vi "add_mppt_data_to_log.vi"(0 "Experiment Indicator":string, 1 "Cell details cluster":T2={"Cell Position"=16, "Cell Label"="", "Pixel to measure"=0, "Area (cm^2)"=0.126, "Variable"="", "Variable value"="", "Scan settings in queue"=0, "Light or dark"="", "Measurement Type"=""} {"Pixel to measure" items=["All", "1", "2", "3", "4", "5", "6", "7", "8"]}, 3 "Intensity (no. of suns)":string, 4 "mppt folder path":path, 5 "mppt file path":path, 7 "Scan settings":T1={"J-V scan"=TRUE, "Start voltage (V)"=0.0, "End voltage (V)"=0.0, "Step voltage (V)"=1.4, "Scan both directions"=TRUE, "Inverted device structure"=FALSE, "Measurement delay (s)"=10.0, "Measurement speed"=0, "Scan rate (V/s)"=0.0, "Stabilisation time (s)"=0.0, "Stabilisation mode"=0, "Stabilisation value (V or A) "=1.0, "Illumination"=0, "Stabilisation in the dark?"=FALSE, "Repeat light scans"=FALSE, "No. of repeat scans"=0.0, "Only repeat for best pixel"=1, "J-t scan"=FALSE, "J-t best pixel only"=7, "J-t start voltage (V)"=0.0, "J-t end voltage (V)"=1.4, "J-t step voltage (V)"=0.01, "Step time (s)"=0.7, "J-t scan both directions"=TRUE, "J-t inverted device structure"=FALSE, "Settling delay (s)"=0.0, "J-t measurement speed"=0, "J-t illumination"=2, "Max. power stabilisation"=FALSE, "Max power best pixel only"=1, "Max. power point tracker"=FALSE, "Vmp from J-V scan"=FALSE, "Max P stab. Specific voltage"=FALSE, "Vmp (V)"=1.0, "Stabilisation time step (s)"=1.0, "Total stabilisation time (s)"=100.0} {"Settling delay (s)" min=0.0; "J-t illumination" items=["Light only", "Dark only", "Light then dark", "Dark then light"]; "Measurement speed" items=["Fast", "Normal", "High accuracy"]; "Illumination" items=["Light only", "Dark only", "Light then dark", "Dark then light"]; "Only repeat for best pixel" items=["only for best pixel", "for best 2 pixels", "for best 3 pixels", "for best 4 pixels", "for best 5 pixels", "for best 6 pixels", "for best 7 pixels", "for all pixels"]; "No. of repeat scans" min=1.0 step=1.0; "Max power best pixel only" items=["only the best pixel", "the best 2 pixels", "the best 3 pixels", "the best 4 pixels", "the best 5 pixels", "the best 6 pixels", "the best 7 pixels", "all pixels"]; "J-t best pixel only" items=["only the best pixel", "the best 2 pixels", "the best 3 pixels", "the best 4 pixels", "the best 5 pixels", "the best 6 pixels", "the best 7 pixels", "all pixels"]; "J-t measurement speed" items=["Fast", "Normal", "High Accuracy"]; "Stabilisation mode" items=["V", "I"]; "Measurement delay (s)" min=0.01}) -> (14 "Master Log":string[][](table), 15 "File path for master log":path)   [LabVIEW 2016]
uses:
  TypeDefs/scan_settings.ctl
  <vilib>/Utility/file.llb/Write To Spreadsheet File (string).vi
  <vilib>/Utility/file.llb/Read From Spreadsheet File (string).vi
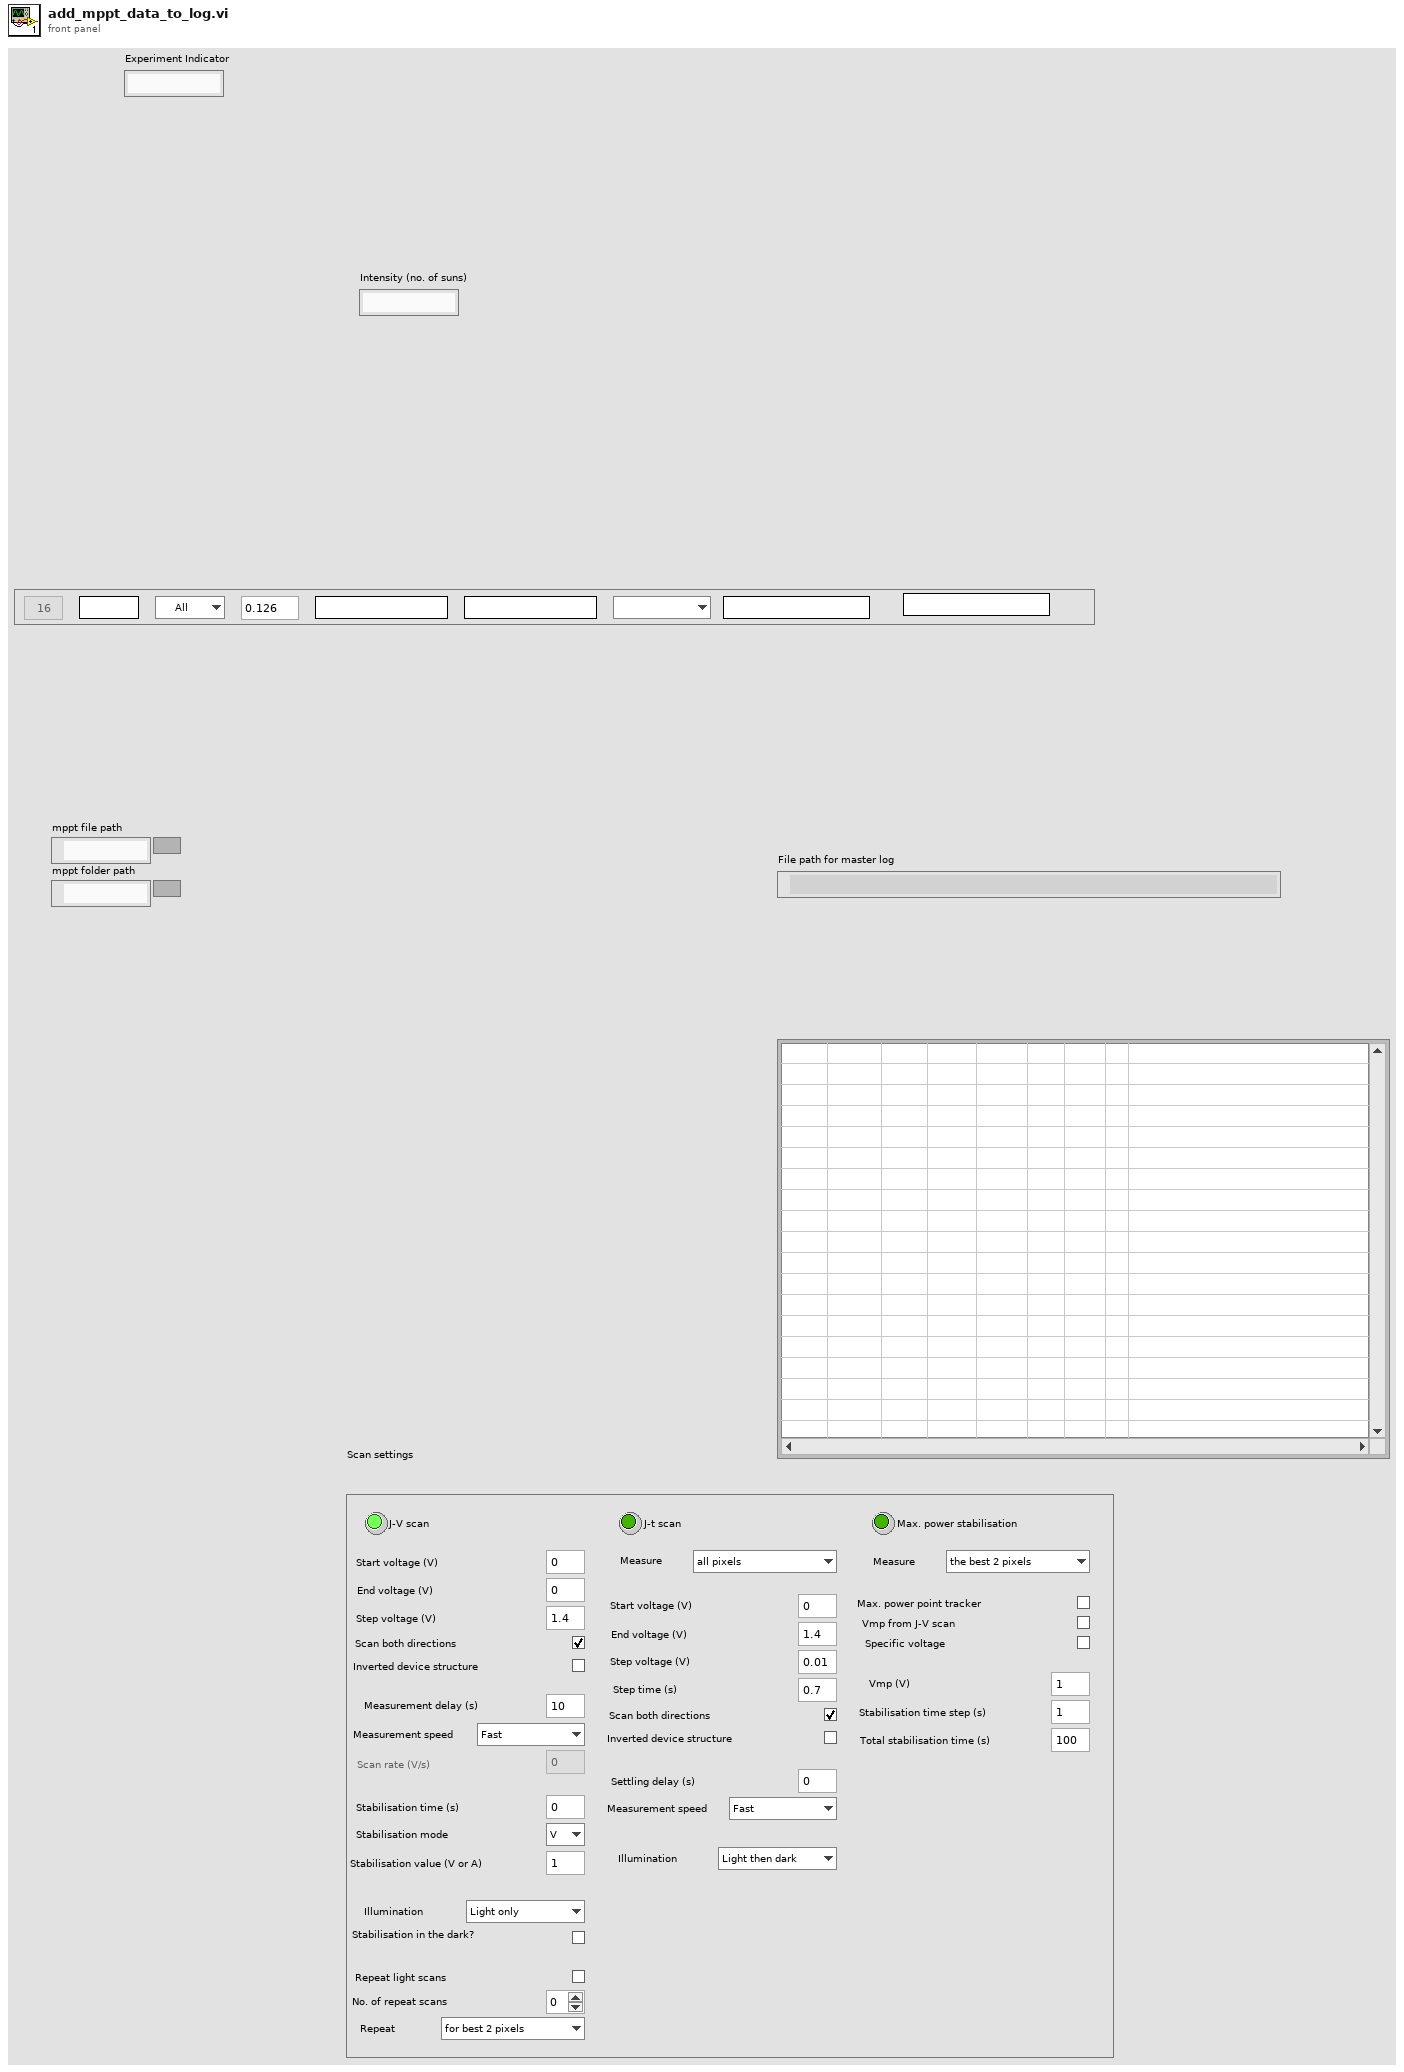
[diagram p1: front panel]
types:
  T1 = typedef "scan_settings.ctl" = cluster{"J-V scan":bool, "Start voltage (V)":dbl, "End voltage (V)":dbl, "Step voltage (V)":dbl, "Scan both directions":bool, "Inverted device structure":bool, "Measurement delay (s)":dbl, "Measurement speed":u8, "Scan rate (V/s)":dbl, "Stabilisation time (s)":dbl, "Stabilisation mode":u16, "Stabilisation value (V or A) ":dbl, "Illumination":u16, "Stabilisation in the dark?":bool, "Repeat light scans":bool, "No. of repeat scans":dbl, "Only repeat for best pixel":u16, "J-t scan":bool, "J-t best pixel only":u16, "J-t start voltage (V)":dbl, "J-t end voltage (V)":dbl, "J-t step voltage (V)":dbl, "Step time (s)":dbl, "J-t scan both directions":bool, "J-t inverted device structure":bool, "Settling delay (s)":dbl, "J-t measurement speed":u16, "J-t illumination":u16, "Max. power stabilisation":bool, "Max power best pixel only":u16, "Max. power point tracker":bool, "Vmp from J-V scan":bool, "Max P stab. Specific voltage":bool, "Vmp (V)":dbl, "Stabilisation time step (s)":dbl, "Total stabilisation time (s)":dbl}
  T2 = cluster{"Cell Position":i32, "Cell Label":string, "Pixel to measure":u16, "Area (cm^2)":dbl, "Variable":string, "Variable value":string, "Scan settings in queue":u16, "Light or dark":string, "Measurement Type":string}
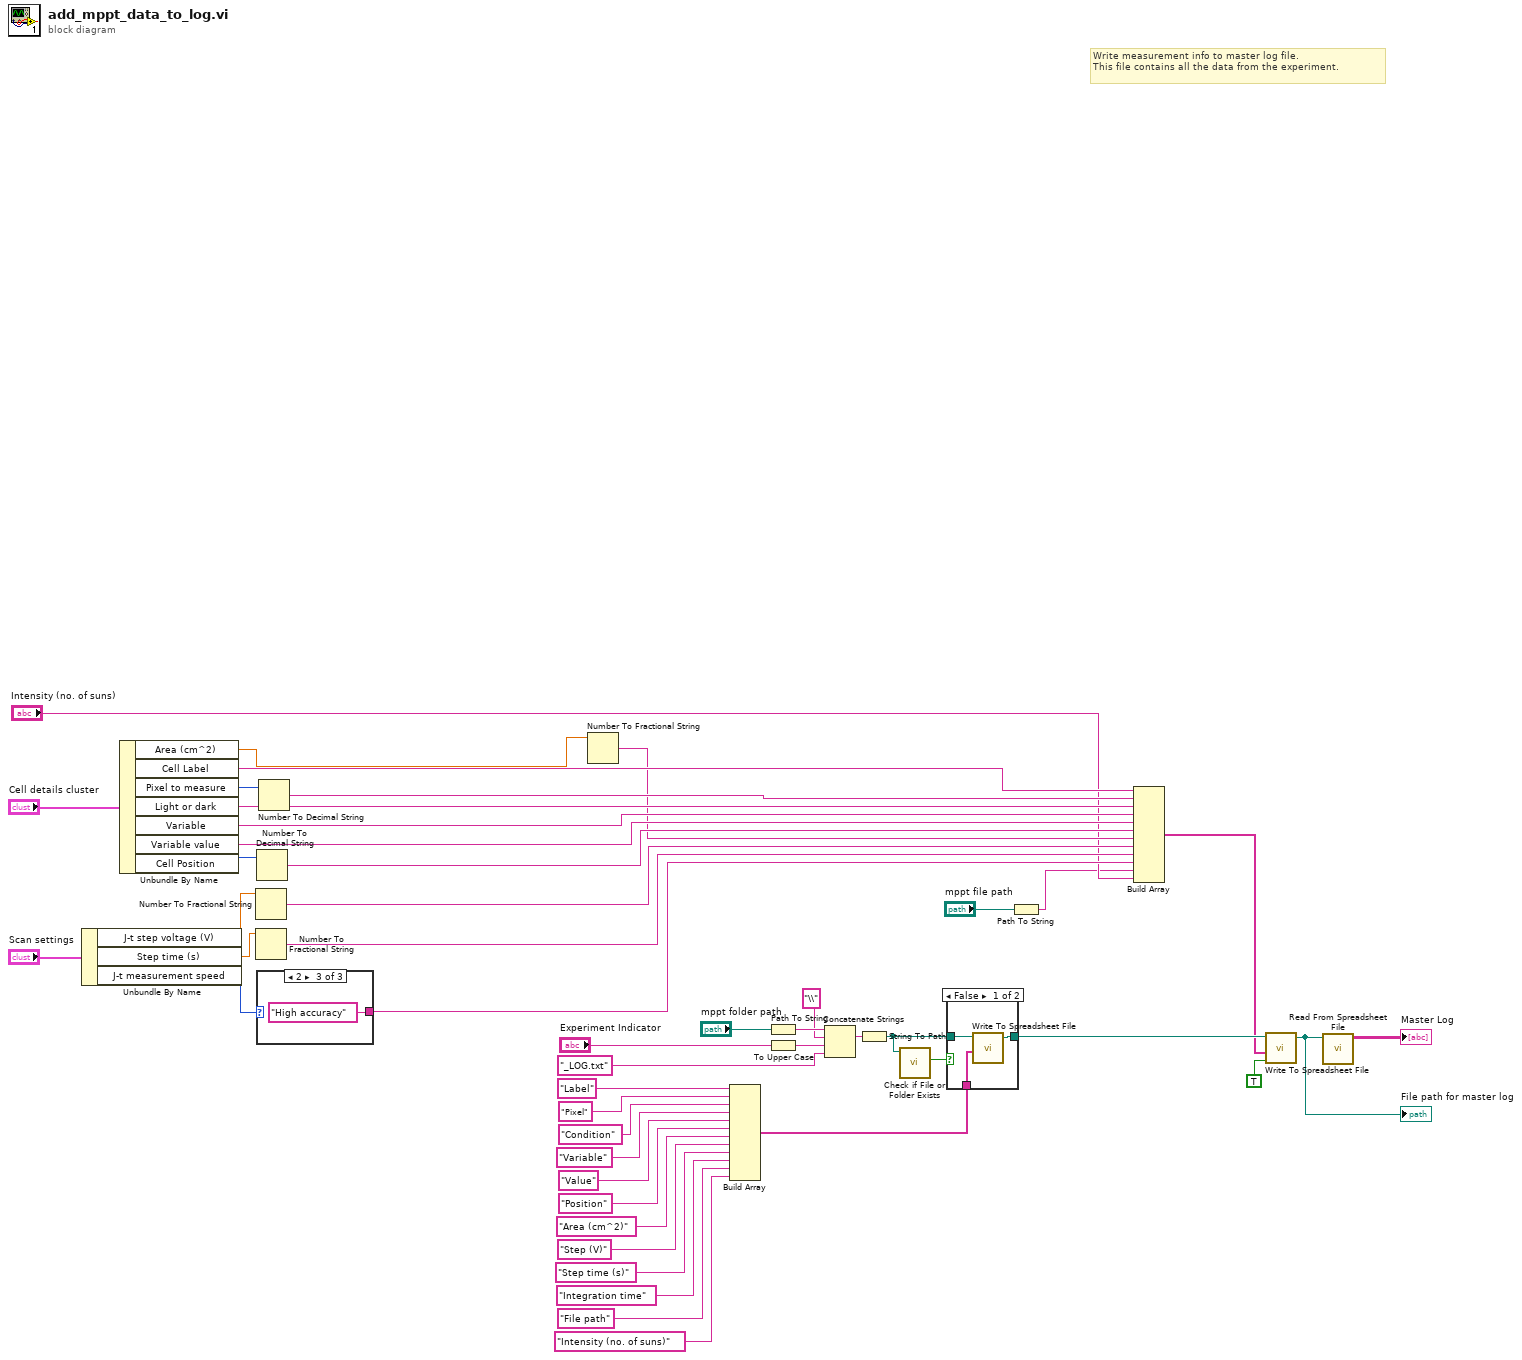
[diagram p0: block diagram]
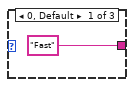
[diagram p2: hidden frame]
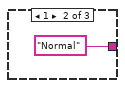
[diagram p3: hidden frame]
diagram:
  # "Write measurement info to master log file.\nThis file contains all the data from the experiment."
  n1 = Unbundle By Name("Scan settings") -> ("J-t step voltage (V)"=w20:dbl, "Step time (s)"=w10:dbl, "J-t measurement speed"=w21:u16)
  n2 = Unbundle By Name("Cell details cluster") -> ("Area (cm^2)"=w12:dbl, "Cell Label"=w19:string, "Pixel to measure"=w47:u16, "Light or dark"=w17:string, "Variable"=w16:string, "Variable value"=w15:string, "Cell Position"=w14:i32)
  n3 = Number To Fractional String(number=w20) -> (F-format string=w9:string)  [unwired: 3 in]
  n4 = Number To Fractional String(number=w10) -> (F-format string=w8:string)  [unwired: 3 in]
  n5 = Number To Decimal String(number=w14) -> (decimal integer string=w13:string)  [unwired: 1 in]
  n6 = case shown="2" w21 {
    tunnel: ["Fast" "Normal" "High accuracy"] -> w7
    frame 0, Default {
    }
    frame 1 {
    }
    frame 2 {
    }
  }
  n7 = Number To Decimal String(number=w47) -> (decimal integer string=w18:string)  [unwired: 1 in]
  n8 = Number To Fractional String(number=w12) -> (F-format string=w11:string)  [unwired: 3 in]
  n9 = Build Array("Label", "Pixel", "Condition", "Variable", "Value", "Position", "Area (cm^2)", "Step (V)", "Step time (s)", "Integration time", "File path", "Intensity (no. of suns)") -> (w23:string[])
  n10 = Path To String(path="mppt folder path") -> (string=w46:string)
  n11 = To Upper Case(1:"Experiment Indicator") -> (0:w39:string)
  n12 = Concatenate Strings(w46, "\\", w39, "_LOG.txt") -> (w44:string)
  n13 = String To Path(string=w44) -> (path=w37:path)
  n14 = call <vilib>:"Check if File or Folder Exists.vi"("path"=w37) -> ("file or folder exists?"=w38:bool)  [unwired: 8 in, 2 out]
  n15 = case shown="False" w38 {
    tunnel: w37 -> [w54 w55]
    tunnel: [w53 w55] -> w36
    tunnel: w23 -> [w52 _]
    frame False {
      n16 = call-poly <vilib>:"Write To Spreadsheet File.vi"("1D data"=w52, "file path (dialog if empty)"=w54) -> ("new file path (Not A Path if cancelled)"=w53:path)  [unwired: 6 in]
    }
    frame True {
    }
  }
  n17 = Path To String(path="mppt file path") -> (string=w4:string)
  n18 = Build Array(w19, w18, w17, w16, w15, w13, w11, w9, w8, w7, w4, "Intensity (no. of suns)") -> (w5:string[])
  n19 = call-poly <vilib>:"Write To Spreadsheet File.vi"("append to file? (new file:F)"=TRUE, "1D data"=w5, "file path (dialog if empty)"=w36) -> ("new file path (Not A Path if cancelled)"=w41:path)  [unwired: 5 in]
  "File path for master log" <- w41
  n20 = call-poly <vilib>:"Read From Spreadsheet File.vi"("file path (dialog if empty)"=w41) -> ("all rows"=→"Master Log":string[][])  [unwired: 6 in, 4 out]
